vi "SDSU_ReadDACS.vi"(7 "fd":i32, 8 "error in (no error)":errorcluster, 9 "argument":string, 10 "action":T1(ring), 11 "file path":path=path "/home/arcconfig/DHE_DACS.cfg") -> (0 "error out":errorcluster, 1 "response":string, 2 "Table":string[][](table), 3 "file path out":path=path "/home/ArcVIEW/ConfigFiles/PI_laboratory.cfg", 5 "index":i32, 6 "fd out":i32)   [LabVIEW 2016]
panel:
  out "resolutions":string[][](array[string])
  in  "current index":u8=6
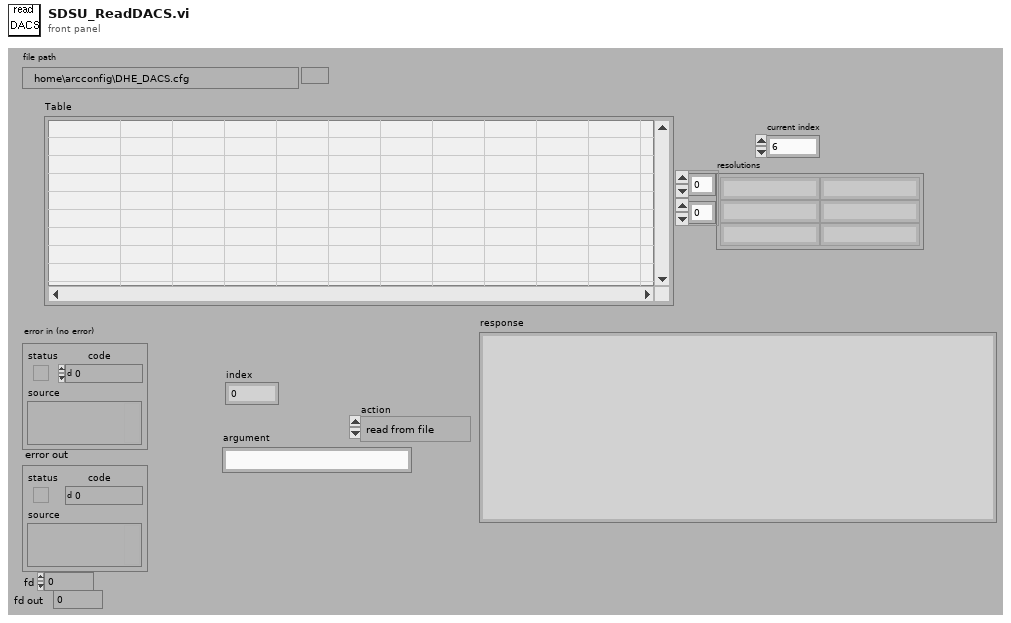
[diagram p1: front panel]
types:
  T1 = enum16{"read from file", "find", "set", "set_to_default", "get all", "resend_last"}
  T2 = typedef "DatabaseHand_RefNum.ctl" = refnum<vi>
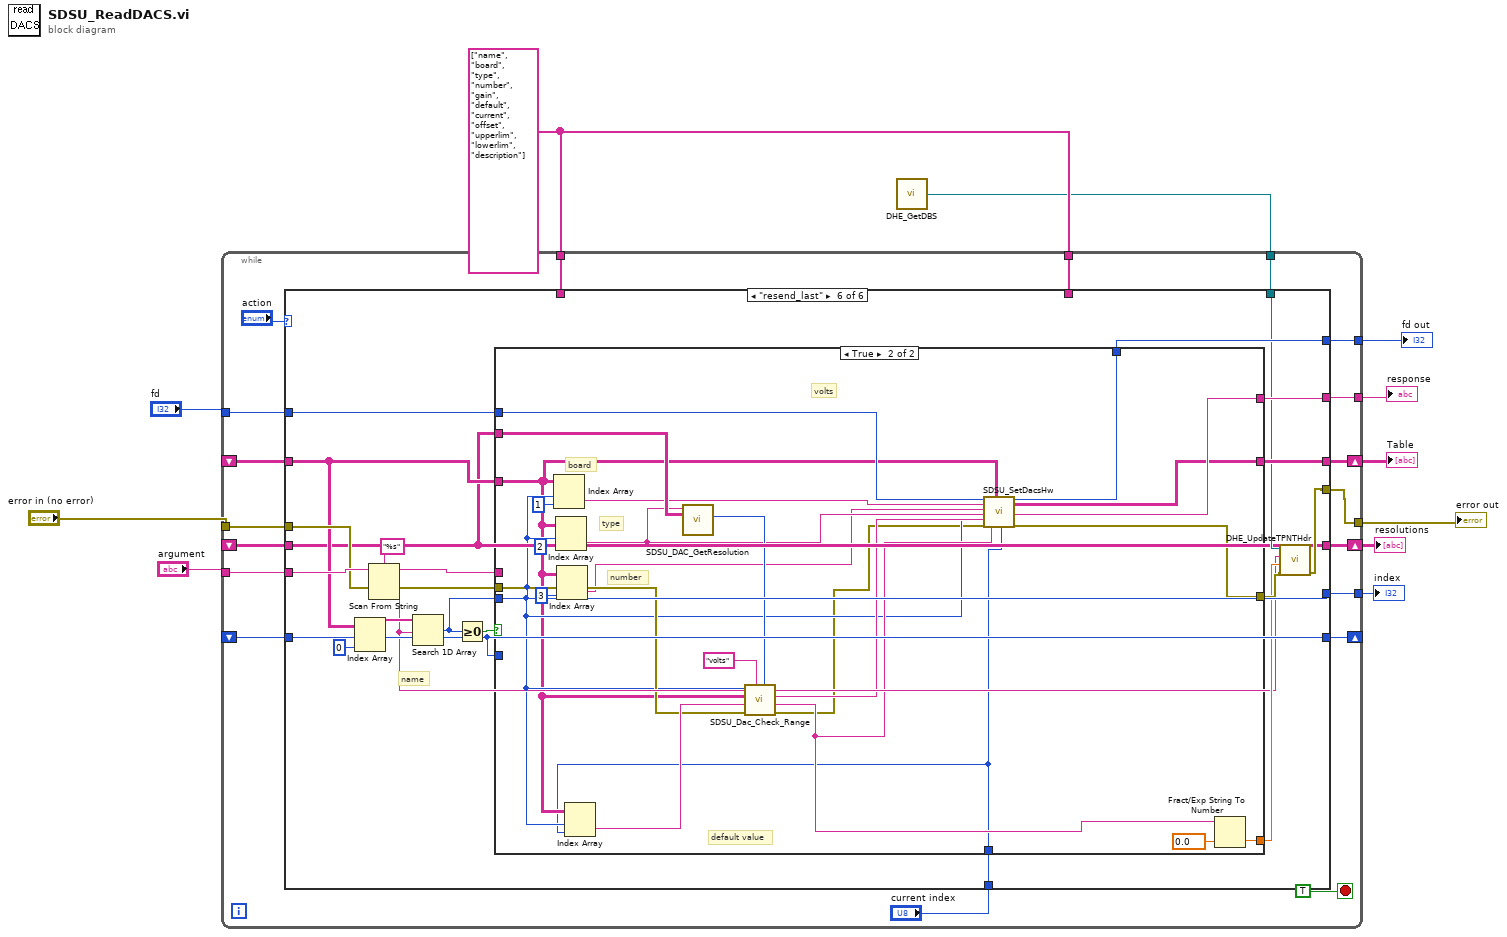
[diagram p0: block diagram]
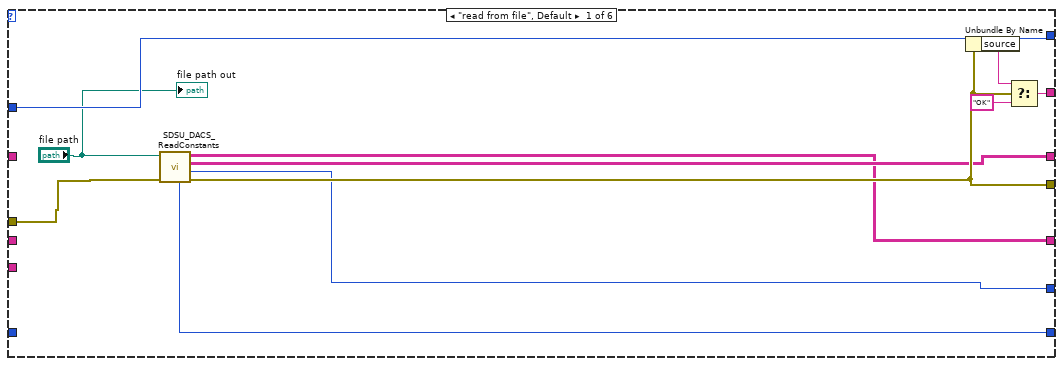
[diagram p2: hidden frame]
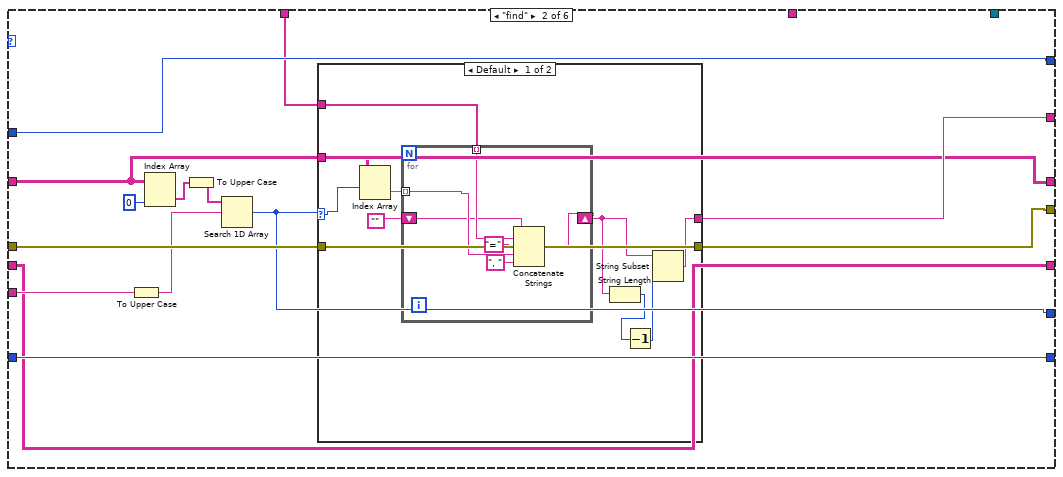
[diagram p3: hidden frame]
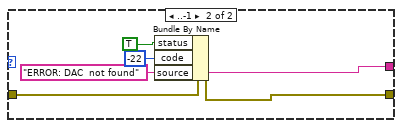
[diagram p4: hidden frame]
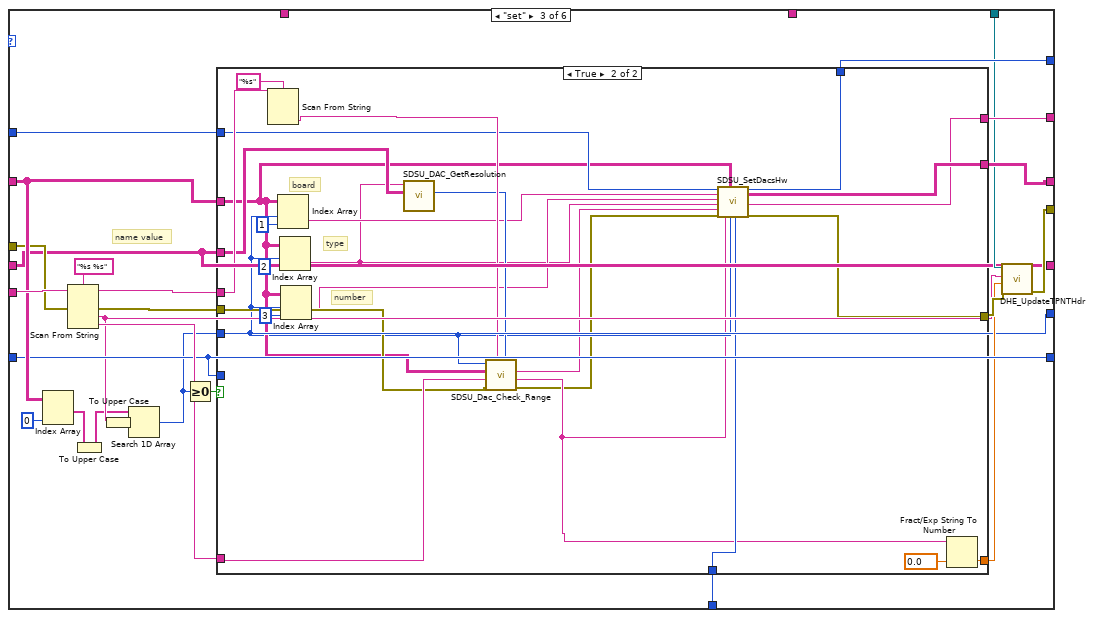
[diagram p5: hidden frame]
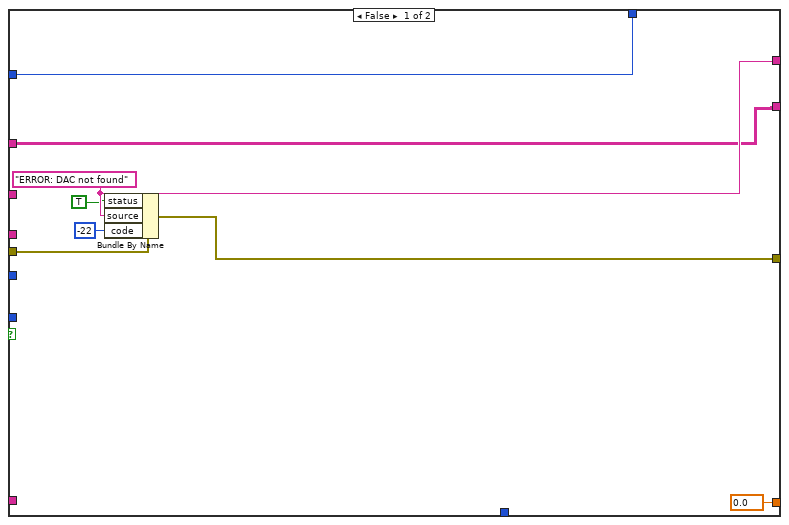
[diagram p6: hidden frame]
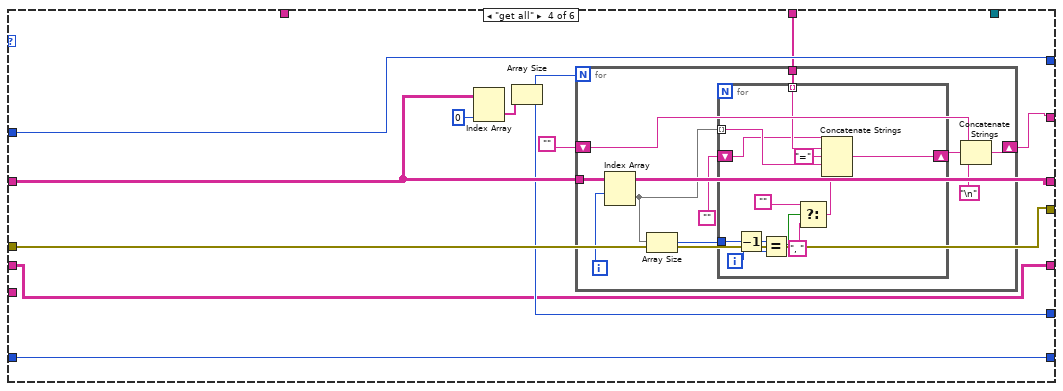
[diagram p7: hidden frame]
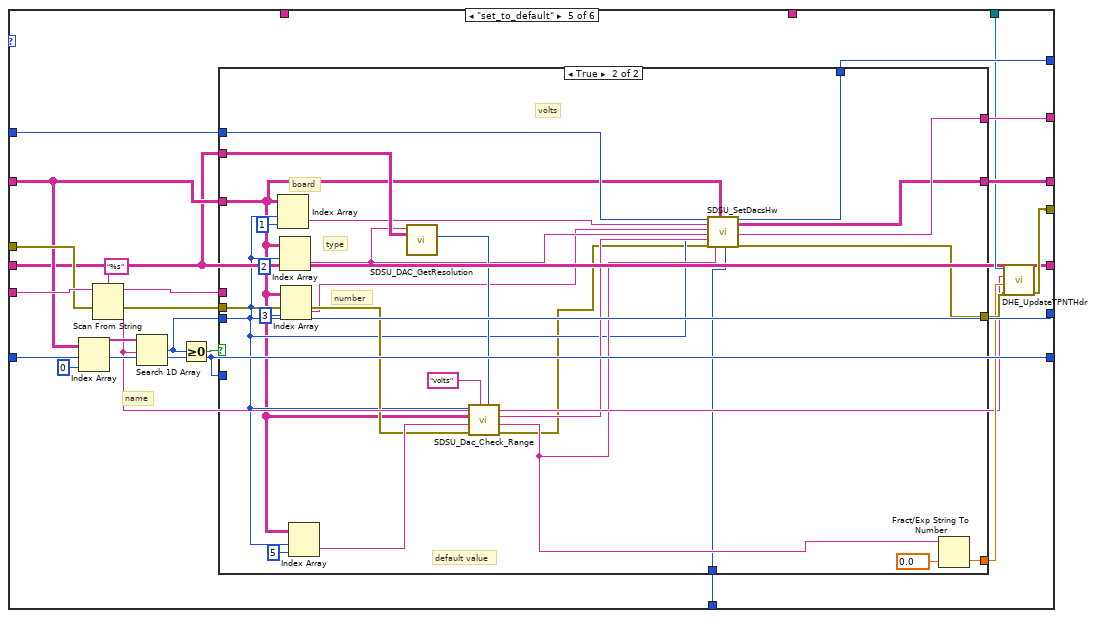
[diagram p8: hidden frame]
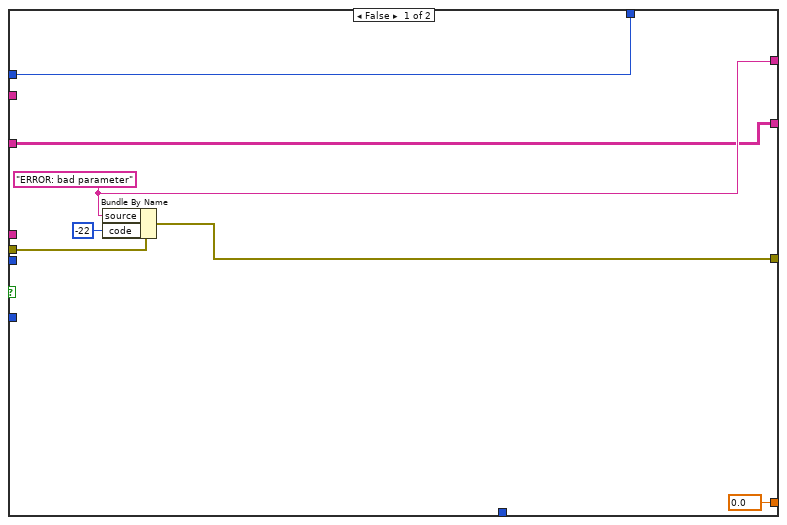
[diagram p9: hidden frame]
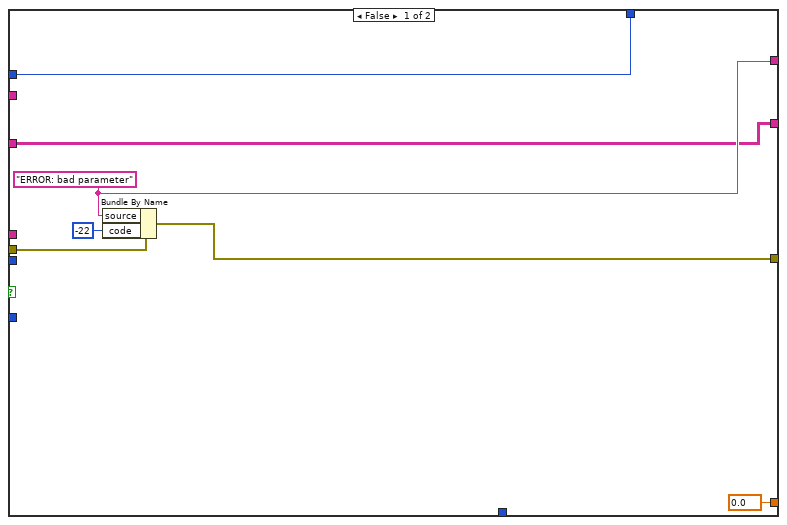
[diagram p10: hidden frame]
diagram:
  w4 = string[] ["name", "board", "type", "number", "gain", "default", "current", "offset", "upperlim", "lowerlim", "description"]
  n1 = call "DHE_GetDBS.vi"() -> ("DHE_DBSRef"=w2:T2)  [unwired: 9 out]
  n2 = while {
    shift-right: [w29] -> w10
    shift-left: _ -> [w25]
    tunnel: "error in (no error)" -> [w28]
    tunnel: [w27] -> w3
    tunnel: [w24] -> w9
    tunnel: "argument" -> [w23]
    tunnel: "fd" -> [w22]
    tunnel: [w21] -> w6
    tunnel: [w18] -> w5
    tunnel: w4 -> [w20]
    tunnel: w4 -> [w19]
    shift-right: [w16] -> _
    shift-left: _ -> [w15]
    tunnel: w2 -> [w14]
    shift-right: [w13] -> w1
    shift-left: _ -> [w12]
    stop <- TRUE stop-if-true
    n3 = case shown="\"resend_last\"" "action" {
      tunnel: [w34 w50 w89 w140 w177 w231] -> w29
      tunnel: w28 -> [w37 w53 w91 w141 w187 w241]
      tunnel: [w35 w52 w85 w141 w172 w226] -> w27
      tunnel: w25 -> [_ w50 w93 w140 w176 w230]
      tunnel: [w39 w51 w94 w138 w183 w237] -> w24
      tunnel: w23 -> [_ w54 w100 _ w189 w243]
      tunnel: w22 -> [w38 w49 w97 w143 w185 w239]
      tunnel: [w38 w49 w96 w143 w184 w238] -> w21
      tunnel: w20 -> [_ w48 _ _ _ _]
      tunnel: w19 -> [_ _ _ w142 _ _]
      tunnel: [w33 w47 w77 w137 w178 w232] -> w18
      tunnel: "current index" -> [_ _ w88 _ w175 w229]
      tunnel: [w32 w46 w87 w136 w174 w228] -> w16
      tunnel: w15 -> [_ w46 w87 w136 w174 w228]
      tunnel: w14 -> [_ _ w82 _ w171 w225]
      tunnel: [w31 w45 w81 w135 w168 w222] -> w13
      tunnel: w12 -> [_ w45 w81 w135 w168 w222]
      frame "read from file", Default {
        n4 = call "SDSU_DACS_ReadConstants.vi"("error in (no error)"=w37, "file path"="file path") -> ("error out"=w35:errorcluster, "number of dacs"=w33:i32, "constants"=w34:string[][], "resolutions"=w31:string[][], "resolution"=w32:i32)  [unwired: 5 out]
        n5 = Unbundle By Name(w35) -> ("source"=w41:string)
        n6 = Select(t=w41, s=w35, f="OK") -> (s? t:f=w39:string)
        "file path out" <- "file path"
      }
      frame "find" {
        n7 = To Upper Case(1:w54) -> (0:w42:string)
        n8 = Index Array(array=w50, index (col)=0 ("disabled index (col)")) -> (element=w44:string[])  [unwired: 1 in]
        n9 = To Upper Case(1:w44) -> (0:w43:string[])
        n10 = Search 1D Array(1D array=w43, element=w42) -> (index of element=w47:i32)  [unwired: 1 out]
        n11 = case shown="Default" w47 {
          selector: w47 -> [w63 _]
          tunnel: w50 -> [w64 _]
          tunnel: w53 -> [w65 w76]
          tunnel: [w65 w75] -> w52
          tunnel: w48 -> [w61 _]
          tunnel: [w57 w72] -> w51
          frame Default {
            n12 = Index Array(array=w64, index (row)=w63) -> (element=w62:string[])  [unwired: 1 in]
            n13 = for {
              tunnel: w62 -> [w71] mode=indexing
              tunnel: w61 -> [w70] mode=indexing
              shift-right: [w69] -> w58
              shift-left: "" -> [w68]
              n14 = Concatenate Strings(w68, w70, "=" ("string"), w71, ", " ("string")) -> (w69:string)
            }
            n15 = String Length(string=w58) -> (length=w59:i32)
            n16 = Decrement(x=w59) -> (x-1=w56:i32)
            n17 = String Subset(string=w58, length (rest)=w56) -> (substring=w57:string)  [unwired: 1 out]
          }
          frame ..-1 {
            w72 = "ERROR: DAC  not found" ("source")
            n18 = Bundle By Name(cluster=w76, "status"=TRUE, "code"=-22, "source"=w72) -> (w75:errorcluster)
          }
        }
      }
      frame "set" {
        # "name value"
        n19 = Index Array(array=w93, index (col)=0 ("disabled index (col)")) -> (element=w80:string[])  [unwired: 1 in]
        n20 = Scan From String(format string="%s %s", input string=w100, error in=w91) -> (remaining string=w98:string, output 1=w84:string, output 2=w95:string)  [unwired: 1 in, 4 out]
        n21 = To Upper Case(1:w80) -> (0:w79:string[])
        n22 = To Upper Case(1:w84) -> (0:w78:string)
        n23 = Search 1D Array(1D array=w79, element=w78) -> (index of element=w77:i32)  [unwired: 1 out]
        n24 = Greater Or Equal To 0?(x=w77) -> (x >= 0?=w90:bool)
        n25 = case shown="True" w90 {
          tunnel: [w107 w109] -> w86
          tunnel: w77 -> [_ w120]
          tunnel: w98 -> [_ w131]
          tunnel: w93 -> [w103 w121]
          tunnel: w97 -> [w106 w122]
          tunnel: [w106 w111] -> w96
          tunnel: w95 -> [_ w129]
          tunnel: [w105 w110] -> w94
          tunnel: w91 -> [w104 w128]
          tunnel: [w103 w112] -> w89
          tunnel: w88 -> [_ w119]
          tunnel: w87 -> [_ _]
          tunnel: [0.0 w126] -> w83
          tunnel: w81 -> [_ w124]
          frame False {
            w105 = "ERROR: DAC not found" ("source")
            n26 = Bundle By Name(cluster=w104, "status"=TRUE, "source"=w105, "code"=-22) -> (w107:errorcluster)
          }
          frame True {
            # "number"
            # "type"
            # "board"
            n27 = Scan From String(format string="%s", input string=w131) -> (output 1=w127:string)  [unwired: 2 in, 4 out]
            n28 = Index Array(array=w121, index (row)=w120, index (col)=1 ("disabled index (col)")) -> (element=w118:string)
            n29 = Index Array(array=w121, index (row)=w120, index (col)=2 ("disabled index (col)")) -> (element=w116:string)
            n30 = Index Array(array=w121, index (row)=w120, index (col)=3 ("disabled index (col)")) -> (element=w117:string)
            n31 = call "SDSU_DAC_GetResolution.vi"("resolutions"=w124, "type"=w116) -> ("max counts"=w123:i32)  [unwired: 9 out]
            n32 = call "SDSU_Dac_Check_Range.vi"("resolution"=w123, "unit"=w127, "error in (no error)"=w128, "value in"=w129, "DACS"=w121, "dac number"=w120) -> ("error out"=w113:errorcluster, "volts value"=w114:string, "dac value"=w115:string)  [unwired: 3 out]
            n33 = call "SDSU_SetDacsHw.vi"("fd"=w122, "board"=w118, "dac number"=w117, "type"=w116, "dac value"=w115, "error IO"=w113, "volts value"=w114, "dac array"=w121, "index"=w120, "current index"=w119) -> ("fd out"=w111:i32, "dac array out"=w112:string[][], "response"=w110:string, "error IO 2"=w109:errorcluster)  [unwired: 6 in]
            n34 = Fract/Exp String To Number(string=w114, default (0 dbl)=0.0) -> (number=w126:dbl)  [unwired: 3 out]
          }
        }
        n35 = call "DHE_UpdateTPNTHdr.vi"("error in (no error)"=w86, "TP value"=w83, "TP name"=w84, "Database RefNum in"=w82) -> ("error out"=w85:errorcluster)  [unwired: 7 out]
      }
      frame "get all" {
        n36 = Index Array(array=w140, index (col)=0 ("disabled index (col)")) -> (element=w144:string[])  [unwired: 1 in]
        n37 = Array Size(array=w144) -> (size(s)=w137:i32)
        n38 = for {
          N: w137 -> [_]
          tunnel: w142 -> [w155]
          tunnel: w140 -> [w154]
          shift-right: [w151] -> w138
          shift-left: "" -> [w150]
          i -> [w153]
          n39 = Index Array(array=w154, index (row)=w153) -> (element=w148:string[])  [unwired: 1 in]
          n40 = Array Size(array=w148) -> (size(s)=w147:i32)
          n41 = for {
            tunnel: w148 -> [w165] mode=indexing
            tunnel: w155 -> [w167] mode=indexing
            shift-right: [w157] -> w146
            shift-left: "" -> [w164]
            tunnel: w147 -> [w162]
            i -> [w163]
            n42 = Decrement(x=w162) -> (x-1=w156:i32)
            n43 = Equal?(x=w156, y=w163) -> (x = y?=w161:bool)
            n44 = Select(t="", s=w161, f=", ") -> (s? t:f=w159:string)
            n45 = Concatenate Strings(w164, w167, "=" ("string"), w165, w159) -> (w157:string)
          }
          n46 = Concatenate Strings(w150, w146, "\n") -> (w151:string)
        }
      }
      frame "set_to_default" {
        # "name"
        n47 = Index Array(array=w176, index (col)=0 ("disabled index (col)")) -> (element=w181:string[])  [unwired: 1 in]
        n48 = Scan From String(format string="%s", input string=w189, error in=w187) -> (remaining string=w186:string, error out=w179:errorcluster, output 1=w169:string)  [unwired: 1 in, 2 out]
        n49 = Search 1D Array(1D array=w181, element=w169) -> (index of element=w178:i32)  [unwired: 1 out]
        n50 = Greater Or Equal To 0?(x=w178) -> (x >= 0?=w180:bool)
        n51 = case shown="True" w180 {
          tunnel: [w195 w200] -> w173
          tunnel: w178 -> [_ w204]
          tunnel: w186 -> [_ _]
          tunnel: w176 -> [w191 w202]
          tunnel: w185 -> [w194 w210]
          tunnel: [w194 w201] -> w184
          tunnel: [w193 w199] -> w183
          tunnel: w179 -> [w192 w215]
          tunnel: [w191 w198] -> w177
          tunnel: w175 -> [_ w203]
          tunnel: w174 -> [_ _]
          tunnel: [0.0 w214] -> w170
          tunnel: w168 -> [_ w212]
          frame False {
            w193 = "ERROR: bad parameter" ("source")
            n52 = Bundle By Name(cluster=w192, "source"=w193, "code"=-22) -> (w195:errorcluster)
          }
          frame True {
            # "default value"
            # "volts"
            # "number"
            # "type"
            # "board"
            n53 = Index Array(array=w202, index (row)=w204, index (col)=1 ("disabled index (col)")) -> (element=w209:string)
            n54 = Index Array(array=w202, index (row)=w204, index (col)=2 ("disabled index (col)")) -> (element=w208:string)
            n55 = Index Array(array=w202, index (row)=w204, index (col)=3 ("disabled index (col)")) -> (element=w207:string)
            n56 = Index Array(array=w202, index (row)=w204, index (col)=5 ("disabled index (col)")) -> (element=w216:string)
            n57 = call "SDSU_DAC_GetResolution.vi"("resolutions"=w212, "type"=w208) -> ("max counts"=w211:i32)  [unwired: 9 out]
            n58 = call "SDSU_Dac_Check_Range.vi"("resolution"=w211, "unit"="volts", "error in (no error)"=w215, "value in"=w216, "DACS"=w202, "dac number"=w204) -> ("error out"=w197:errorcluster, "volts value"=w205:string, "dac value"=w206:string)  [unwired: 3 out]
            n59 = call "SDSU_SetDacsHw.vi"("fd"=w210, "board"=w209, "dac number"=w207, "type"=w208, "dac value"=w206, "error IO"=w197, "volts value"=w205, "dac array"=w202, "index"=w204, "current index"=w203) -> ("fd out"=w201:i32, "dac array out"=w198:string[][], "response"=w199:string, "error IO 2"=w200:errorcluster)  [unwired: 6 in]
            n60 = Fract/Exp String To Number(string=w205, default (0 dbl)=0.0) -> (number=w214:dbl)  [unwired: 3 out]
          }
        }
        n61 = call "DHE_UpdateTPNTHdr.vi"("error in (no error)"=w173, "TP value"=w170, "TP name"=w169, "Database RefNum in"=w171) -> ("error out"=w172:errorcluster)  [unwired: 7 out]
      }
      frame "resend_last" {
        # "name"
        n62 = Index Array(array=w230, index (col)=0 ("disabled index (col)")) -> (element=w235:string[])  [unwired: 1 in]
        n63 = Scan From String(format string="%s", input string=w243, error in=w241) -> (remaining string=w240:string, error out=w233:errorcluster, output 1=w223:string)  [unwired: 1 in, 2 out]
        n64 = Search 1D Array(1D array=w235, element=w223) -> (index of element=w232:i32)  [unwired: 1 out]
        n65 = Greater Or Equal To 0?(x=w232) -> (x >= 0?=w234:bool)
        n66 = case shown="True" w234 {
          tunnel: [w249 w255] -> w227
          tunnel: w232 -> [_ w258]
          tunnel: w240 -> [_ _]
          tunnel: w230 -> [w245 w257]
          tunnel: w239 -> [w248 w264]
          tunnel: [w248 w256] -> w238
          tunnel: [w247 w254] -> w237
          tunnel: w233 -> [w246 w269]
          tunnel: [w245 w253] -> w231
          tunnel: w229 -> [_ w251]
          tunnel: w228 -> [_ _]
          tunnel: [0.0 w268] -> w224
          tunnel: w222 -> [_ w266]
          frame False {
            w247 = "ERROR: bad parameter" ("source")
            n67 = Bundle By Name(cluster=w246, "source"=w247, "code"=-22) -> (w249:errorcluster)
          }
          frame True {
            # "default value"
            # "volts"
            # "number"
            # "type"
            # "board"
            n68 = Index Array(array=w257, index (row)=w258, index (col)=1 ("disabled index (col)")) -> (element=w263:string)
            n69 = Index Array(array=w257, index (row)=w258, index (col)=2 ("disabled index (col)")) -> (element=w262:string)
            n70 = Index Array(array=w257, index (row)=w258, index (col)=3 ("disabled index (col)")) -> (element=w261:string)
            n71 = Index Array(array=w257, index (row)=w258, index (col)=w251) -> (element=w270:string)
            n72 = call "SDSU_DAC_GetResolution.vi"("resolutions"=w266, "type"=w262) -> ("max counts"=w265:i32)  [unwired: 9 out]
            n73 = call "SDSU_Dac_Check_Range.vi"("resolution"=w265, "unit"="volts", "error in (no error)"=w269, "value in"=w270, "DACS"=w257, "dac number"=w258) -> ("error out"=w252:errorcluster, "volts value"=w259:string, "dac value"=w260:string)  [unwired: 3 out]
            n74 = call "SDSU_SetDacsHw.vi"("fd"=w264, "board"=w263, "dac number"=w261, "type"=w262, "dac value"=w260, "error IO"=w252, "volts value"=w259, "dac array"=w257, "index"=w258, "current index"=w251) -> ("fd out"=w256:i32, "dac array out"=w253:string[][], "response"=w254:string, "error IO 2"=w255:errorcluster)  [unwired: 6 in]
            n75 = Fract/Exp String To Number(string=w259, default (0 dbl)=0.0) -> (number=w268:dbl)  [unwired: 3 out]
          }
        }
        n76 = call "DHE_UpdateTPNTHdr.vi"("error in (no error)"=w227, "TP value"=w224, "TP name"=w223, "Database RefNum in"=w225) -> ("error out"=w226:errorcluster)  [unwired: 7 out]
      }
    }
  }
  "error out" <- w3
  "Table" <- w10
  "response" <- w9
  "fd out" <- w6
  "index" <- w5
  "resolutions" <- w1
